vi "SaveCsvDATE_Hid.vi"() -> (2 "输出数组":string[][](array[string]))   [LabVIEW 2018]
uses:
  Subvi/Global.vi
panel:
  out "数组":string[](array[string])
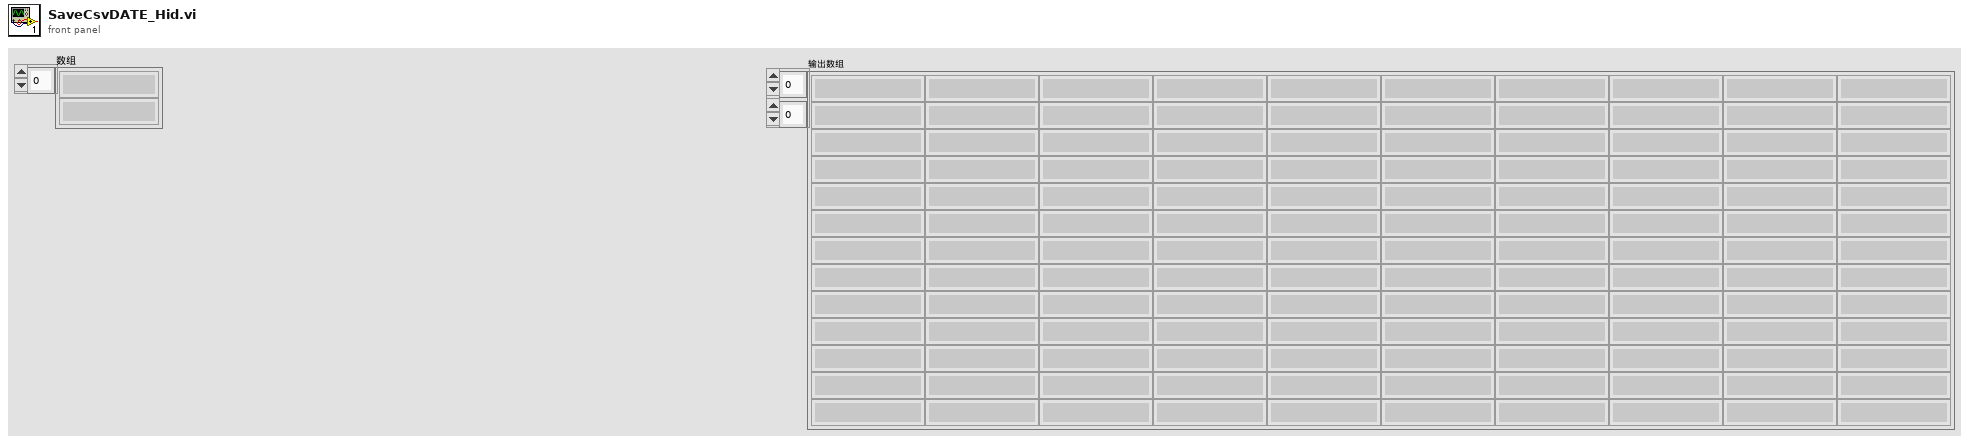
[diagram p1: front panel]
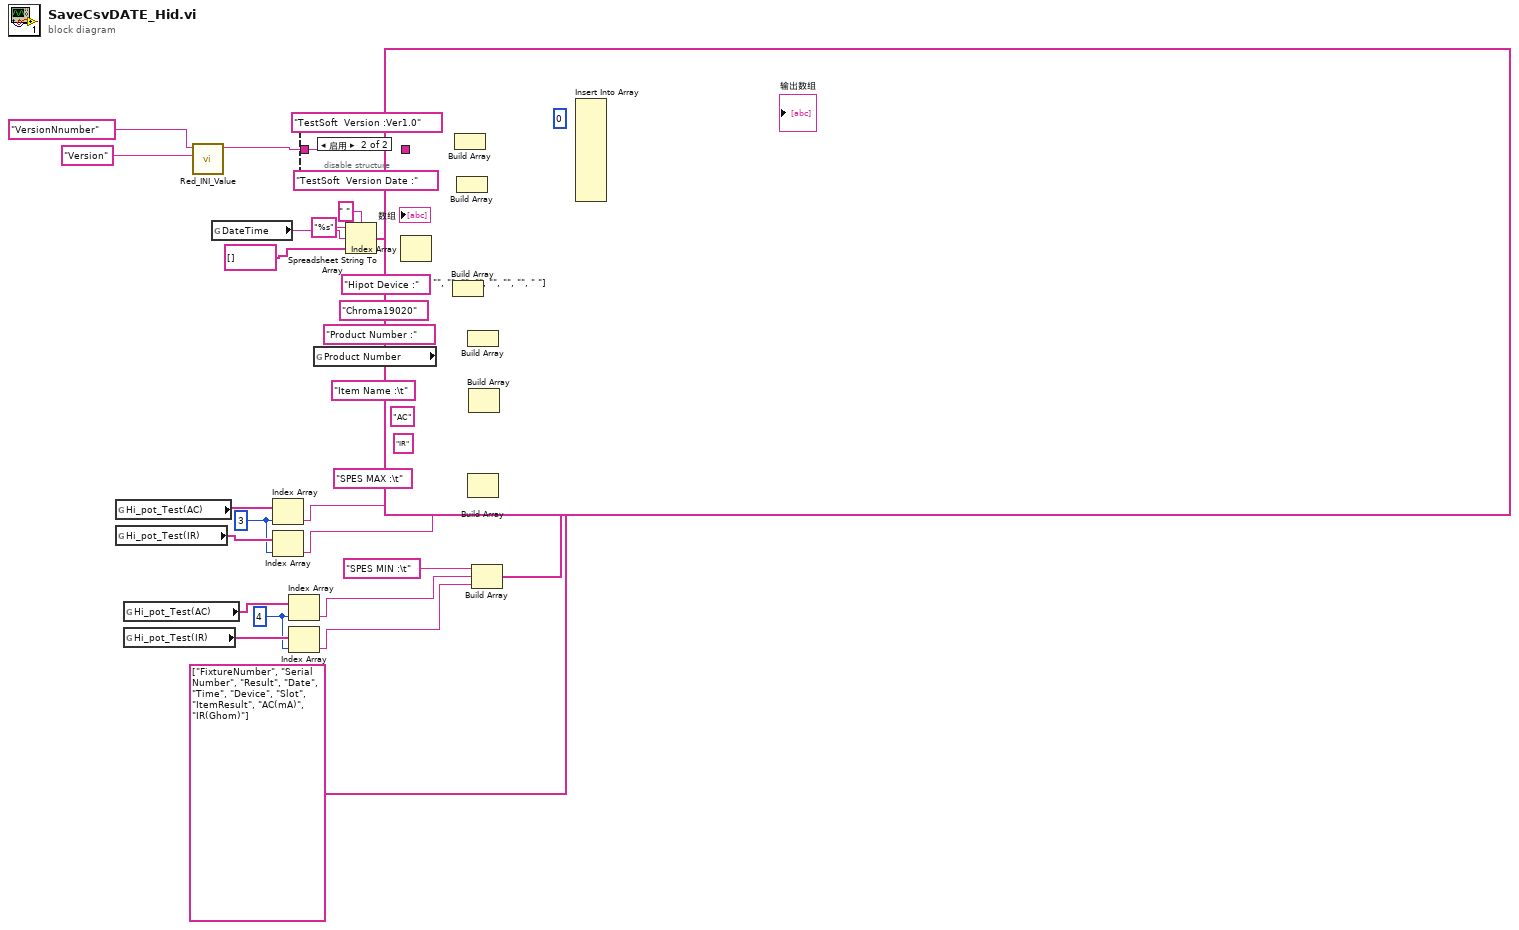
[diagram p0: block diagram]
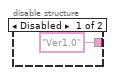
[diagram p2: hidden frame]
diagram:
  w3 = 4 ("索引")
  w8 = 3 ("索引")
  n1 = global read "Global.vi" "Hi_pot_Test(AC)"() -> (w10:string[])
  n2 = global read "Global.vi" "Hi_pot_Test(IR)"() -> (w9:string[])
  n3 = global read "Global.vi" "Hi_pot_Test(AC)"() -> (w5:string[])
  n4 = global read "Global.vi" "Hi_pot_Test(IR)"() -> (w4:string[])
  n5 = call "Red_INI_Value.vi"("section"="Version", "section 2"="VersionNnumber" ("section")) -> ("value"=w11:string)  [unwired: 9 in]
  n6 = global read "Global.vi" "DateTime"() -> (w36:string)
  n7 = Index Array(array=w10, index=w8) -> (element=w7:string)
  n8 = Index Array(array=w9, index=w8) -> (element=w6:string)
  n9 = Index Array(array=w5, index=w3) -> (element=w2:string)
  n10 = Index Array(array=w4, index=w3) -> (element=w1:string)
  n11 = disable-structure shown="启用" {
    disable-tunnel: ["Ver1.0" w44] -> w15
    disable-tunnel: w11 -> [_ w44]
    frame Disabled {
    }
    frame Enabled {
    }
  }
  n12 = global read "Global.vi" "Product Number"() -> (w38:string)
  n13 = Spreadsheet String To Array(delimiter (Tab)=" " ("分隔符(Tab)"), format string="%s" ("格式字符串"), spreadsheet string=w36, array type (2D Dbl)=string[] []) -> (array=w31:string[])
  "数组" <- w31
  n14 = Index Array(array=w31) -> (element=w29:string)  [unwired: 1 in]
  n15 = Build Array("Hipot Device :", "Chroma19020") -> (w27:string[])
  n16 = Build Array("TestSoft  Version :Ver1.0", w15) -> (w40:string[])
  n17 = Build Array("TestSoft  Version Date :", w29) -> (w28:string[])
  n18 = Build Array("Product Number :", w38) -> (w26:string[])
  n19 = Build Array("SPES MAX :\t", w7, w6) -> (w20:string[])
  n20 = Build Array("Item Name :\t", "AC", "IR") -> (w21:string[])
  n21 = Build Array("SPES MIN :\t", w2, w1) -> (w16:string[])
  n22 = Insert Into Array(array=string[][] [["", "", "", "", "", "", "", "", "", "", " "]], index (row)=0 ("索引 (行)"), new element #1=w40, new element #2=w28, new element #3=w27, new element #4=w26, new element #5=w21, new element #6=w20, new element #7=w16, new element #8=string[] ["FixtureNumber", "Serial Number", "Result", "Date", "Time", "Device", "Slot", "ItemResult", "AC(mA)", "IR(Ghom)"]) -> (→"输出数组":string[][])  [unwired: 1 in]
